vi "JoysticksGlobal.vi"() -> ()   [LabVIEW 2019]
panel:
  out "RT":dbl
  out "LT":dbl
  out "AutoAxe4":dbl
  out "AutoAxe1":dbl
  out "Button 0":bool
  out "Button 2":bool
  out "Rumble":dbl
  out "Button 7":bool
  out "Button 6":bool
  out "OpAxe 4":dbl
  out "OpRT":dbl
  out "OpLT":dbl
  in  "DpadLeft":bool
  in  "DpadDown":bool
  in  "DpadUP":bool
  out "OpButton 5":bool
  out "OpButton 4":bool
  out "OpButton 3":bool
  out "OpButton 2":bool
  out "OpButton 1":bool
  out "OpButton 0":bool
  out "Button 5":bool
  out "Button 4":bool
  out "Axe 4":dbl
  out "Axe 1":dbl
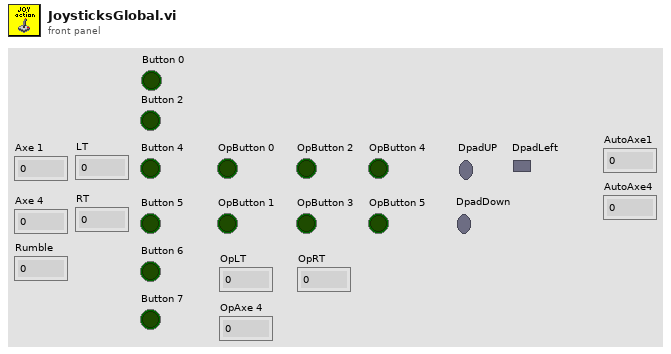
[diagram p1: front panel]
diagram:
